vi "PumpModeSet.vi"(8 "Error In":errorcluster, 9 "Pump Mode":T1=2 items=["Drain", "Fill", "Normal"], 10 "delay before read (ms)":u32=500, 11 "VISA resource name":refnum<visa-resource-name>="COM7") -> (0 "Error Out":errorcluster, 1 "Write byte count":u32, 2 "Read byte count":u32, 3 "read buffer":string)   [LabVIEW 2016]
uses:
  PumpModeSelector.ctl
  <vilib>/Instr/_visa.llb/VISA Configure Serial Port (Instr).vi
panel:
  out "Bytes read":u32
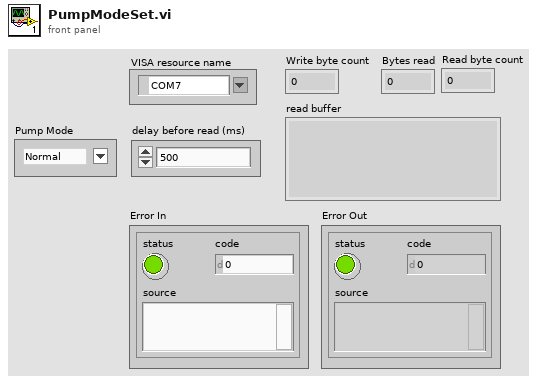
[diagram p1: front panel]
types:
  T1 = typedef "PumpModeSelector.ctl" = u16
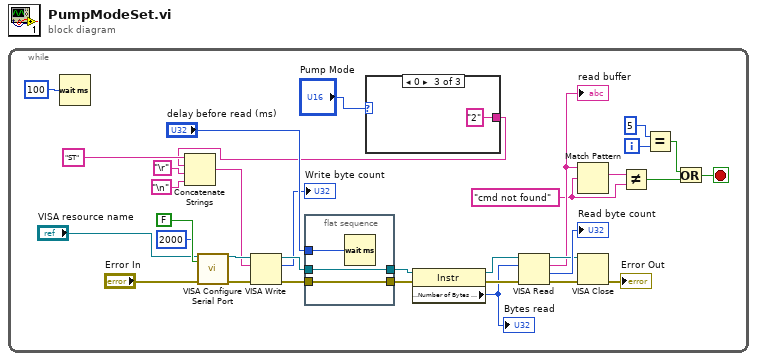
[diagram p0: block diagram]
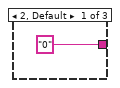
[diagram p2: hidden frame]
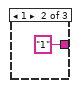
[diagram p3: hidden frame]
diagram:
  n1 = while {
    i -> [w9]
    stop <- w5 stop-if-true
    w10 = "cmd not found" ("regular expression")
    n2 = Wait (ms)(milliseconds to wait=u32 100) -> ()  [unwired: 1 out]
    n3 = call-poly "VISA Configure Serial Port"("VISA resource name"="VISA resource name", "timeout (10sec)"=u32 2000, "Enable Termination\nChar (T)"=FALSE ("Enable Termination\nChar (T)"), "error in (no error)"="Error In") -> ("VISA resource name out"=w30:refnum<visa-resource-name>, "error out"=w28:errorcluster)  [unwired: 5 in, 5 out]
    n4 = flat-sequence {
      tunnel: w25 -> [w39]
      tunnel: [w39] -> w23
      tunnel: w26 -> [w38]
      tunnel: [w38] -> w22
      tunnel: "delay before read (ms)" -> [w40]
      frame #0 {
        n5 = Wait (ms)(milliseconds to wait=w40) -> ()  [unwired: 1 out]
      }
    }
    n6 = case shown="0" "Pump Mode" {
      tunnel: ["0" "1" "2"] -> w1
      frame 2, Default {
      }
      frame 1 {
      }
      frame 0 {
      }
    }
    n7 = Concatenate Strings("ST" ("Command"), w1, "\r", "\n") -> (w29:string)
    n8 = VISA Write(VISA resource name=w30, write buffer=w29, error in (no error)=w28) -> (VISA resource name out=w26:refnum<visa-resource-name>, return count=→"Write byte count":u32, error out=w25:errorcluster)
    n9 = property class="Instr"(reference=w22, error in=w23) -> (reference out=w18:refnum<visa-resource-name>, error out=w17:errorcluster, "Serial Settings:Number of Bytes at Serial Port"=w16:u32)
    "Bytes read" <- w16
    n10 = VISA Read(VISA resource name=w18, byte count=w16, error in (no error)=w17) -> (VISA resource name out=w20:refnum<visa-resource-name>, read buffer=w12:string, return count=→"Read byte count":u32, error out=w19:errorcluster)
    "read buffer" <- w12
    n11 = Match Pattern(string=w12, regular expression=w10) -> (match substring=w11:string)  [unwired: 1 in, 3 out]
    n12 = VISA Close(VISA resource name=w20, error in (no error)=w19) -> (error out=→"Error Out":errorcluster)
    n13 = Not Equal?(x=w11, y=w10) -> (x != y?=w6:bool)
    n14 = Equal?(x=5, y=w9) -> (x = y?=w7:bool)
    n15 = Or(x=w7, y=w6) -> (x .or. y?=w5:bool)
  }
